vi "RILIS Narrow Band Scan Coordinator.vi"() -> ()   [LabVIEW 2013]
uses:
  RILIS Narrow Band Scan Coordinator States.ctl
panel:
  in  "Shared Variable Selection":enum16{"CRIS", "Test"}(ring)
  out "waveReadback":dbl format="%#.4f"
  in  "waveSet":dbl format="%.4f"
  out "Current State":T1
  in  "Find Center":bool
  out "Actual Wavenumber":dbl format="%#.4f"
  out "Loop Counter":i32
  in  "Stop Program":bool
  in  "Scanning Step Size":dbl format="%#.4f"
  in  "End of Scan Range":dbl format="%#.4f"
  in  "Start of Scan Range":dbl format="%#.4f"
  out "Measurement Complete":bool
  out "Averaging Active":bool
  out "isOK":bool
  in  "isNew":bool
  out "Linewidth Sweep Done":bool
  out "Moving to Setpoint":bool
  in  "Setpoint Wavenumber":dbl format="%.4f"
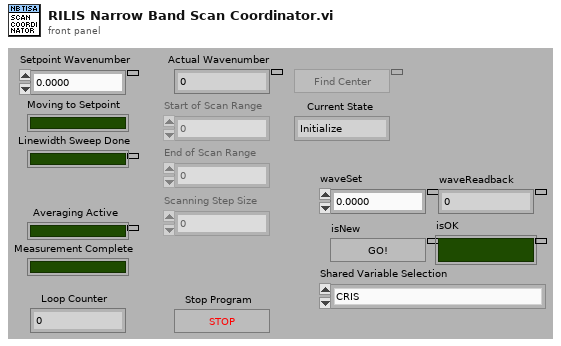
[diagram p1: front panel]
types:
  T1 = typedef "RILIS Narrow Band Scan Coordinator States.ctl" = enum16{"Initialize", "Idle", "Read Setpoint WN", "Check Setpoint WN", "Move to Setpoint WN", "Perform Sweep", "Wait for Ready", "Measurement in Progress", "Stop"}
  T2 = cluster{"Moving to Setpoint":bool, "Linewidth Sweep Done":bool, "Ready to Average":bool, "Averaging Active":bool, "Measurement Complete":bool, "Setpoint Wavenumber":dbl}
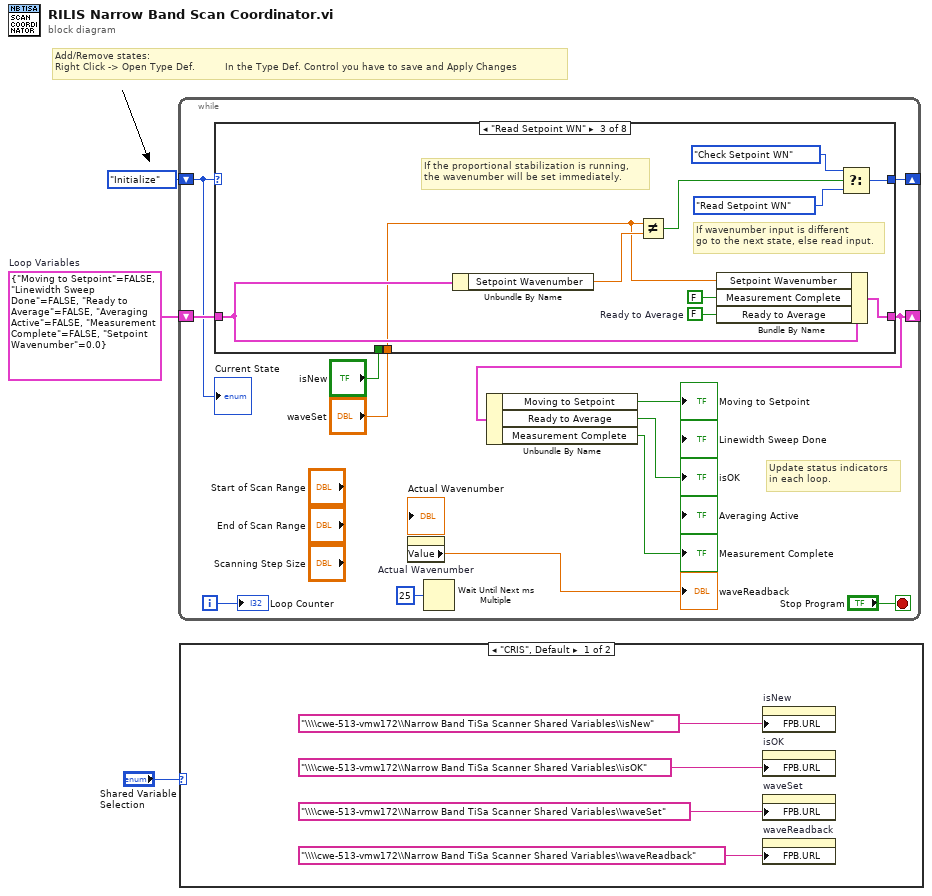
[diagram p0: block diagram]
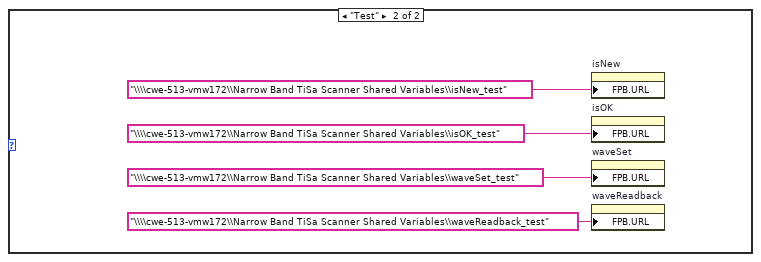
[diagram p2: hidden frame]
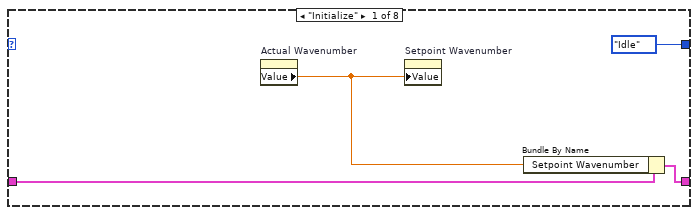
[diagram p3: hidden frame]
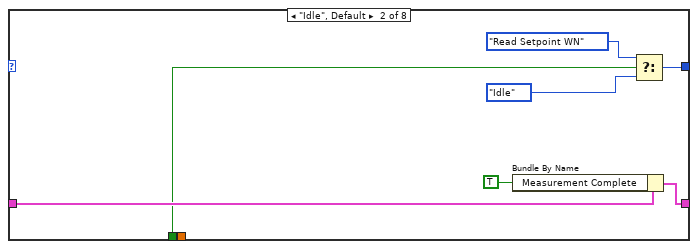
[diagram p4: hidden frame]
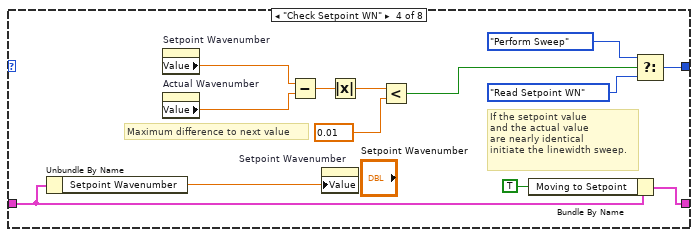
[diagram p5: hidden frame]
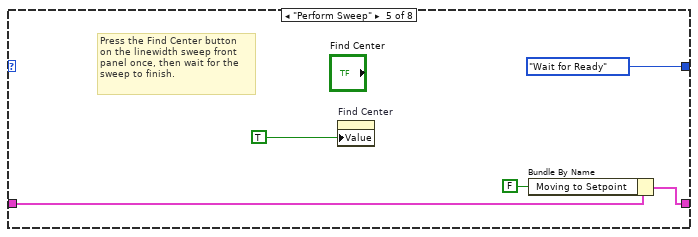
[diagram p6: hidden frame]
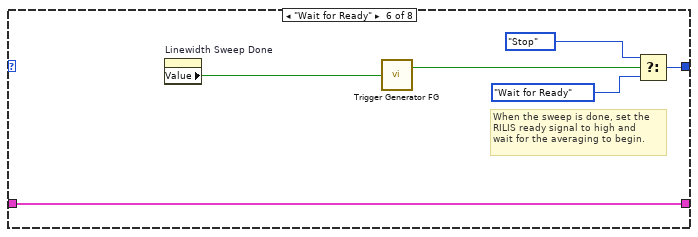
[diagram p7: hidden frame]
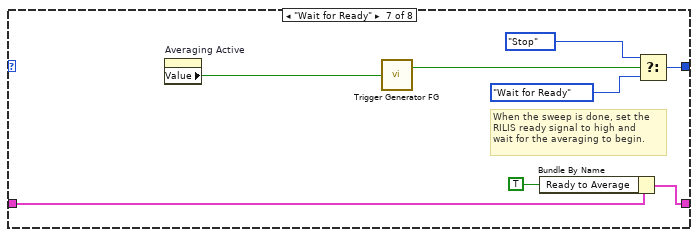
[diagram p8: hidden frame]
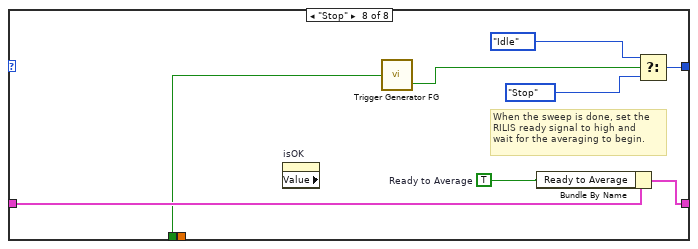
[diagram p9: hidden frame]
diagram:
  w2 = T2 {"Moving to Setpoint"=FALSE, "Linewidth Sweep Done"=FALSE, "Ready to Average"=FALSE, "Averaging Active"=FALSE, "Measurement Complete"=FALSE, "Setpoint Wavenumber"=0.0}  # Loop Variables
  # "Add/Remove states:\nRight Click -> Open Type Def.          In the Type Def. Control you have to save and Apply Changes"
  n1 = while {
    shift-right: [w13] -> _
    shift-left: RILIS_Narrow_Band_Scan_Coordinator_States."Initialize" ("NB Scan States") -> [w11]
    shift-right: [w10] -> _
    shift-left: w2 -> [w12]
    i -> [w15]
    stop <- "Stop Program" stop-if-true
    # "Update status indicators \nin each loop."
    n2 = case shown="\"Read Setpoint WN\"" w11 {
      tunnel: [RILIS_Narrow_Band_Scan_Coordinator_States."Idle" ("NB Scan States") w25 w37 w43 RILIS_Narrow_Band_Scan_Coordinator_States."Wait for Ready" ("NB Scan States") w59 w67 w75] -> w13
      tunnel: w12 -> [w19 w23 w32 w39 w52 w56 w63 w73]
      tunnel: [w18 w22 w31 w41 w51 w56 w62 w72] -> w10
      tunnel: "isNew" -> [_ w21 _ _ _ _ _ w70]
      tunnel: "waveSet" -> [_ _ w29 _ _ _ _ _]
      frame "Initialize" {
        n3 = property on="Actual Wavenumber" class="DigNum (strict)"() -> ("Value"=w17:dbl)  [unwired: 2 in, 2 out]
        n4 = property on="Setpoint Wavenumber" class="DigNum (strict)"("Value"=w17) -> ()  [unwired: 2 in, 2 out]
        n5 = Bundle By Name(cluster=w19, "Setpoint Wavenumber"=w17) -> (w18:T2)
      }
      frame "Idle", Default {
        n6 = Bundle By Name(cluster=w23, "Measurement Complete"=TRUE) -> (w22:T2)
        n7 = Select(t=RILIS_Narrow_Band_Scan_Coordinator_States."Read Setpoint WN" ("NB Scan States"), s=w21, f=RILIS_Narrow_Band_Scan_Coordinator_States."Idle" ("NB Scan States")) -> (s? t:f=w25:T1)
      }
      frame "Read Setpoint WN" {
        w28 = FALSE  # Ready to Average
        # "If wavenumber input is different\ngo to the next state, else read input."
        # "If the proportional stabilization is running, \nthe wavenumber will be set immediately."
        n8 = Unbundle By Name(w32) -> ("Setpoint Wavenumber"=w34:dbl)
        n9 = Not Equal?(x=w29, y=w34) -> (x != y?=w30:bool)
        n10 = Bundle By Name(cluster=w32, "Setpoint Wavenumber"=w29, "Measurement Complete"=FALSE, "Ready to Average"=w28) -> (w31:T2)
        n11 = Select(t=RILIS_Narrow_Band_Scan_Coordinator_States."Check Setpoint WN" ("NB Scan States"), s=w30, f=RILIS_Narrow_Band_Scan_Coordinator_States."Read Setpoint WN" ("NB Scan States")) -> (s? t:f=w37:T1)
      }
      frame "Check Setpoint WN" {
        # "Maximum difference to next value"
        # "If the setpoint value \nand the actual value\nare nearly identical \ninitiate the linewidth sweep."
        n12 = Unbundle By Name(w39) -> ("Setpoint Wavenumber"=w38:dbl)
        n13 = property on="Setpoint Wavenumber" class="DigNum (strict)"() -> ("Value"=w50:dbl)  [unwired: 2 in, 2 out]
        n14 = property on="Actual Wavenumber" class="DigNum (strict)"() -> ("Value"=w49:dbl)  [unwired: 2 in, 2 out]
        n15 = Subtract(x=w50, y=w49) -> (x-y=w48:dbl)
        n16 = property on="Setpoint Wavenumber" class="DigNum (strict)"("Value"=w38) -> ()  [unwired: 2 in, 2 out]
        n17 = Absolute Value(x=w48) -> (abs(x)=w47:dbl)
        n18 = Less?(x=w47, y=0.01) -> (x < y?=w42:bool)
        n19 = Bundle By Name(cluster=w39, "Moving to Setpoint"=TRUE) -> (w41:T2)
        n20 = Select(t=RILIS_Narrow_Band_Scan_Coordinator_States."Perform Sweep" ("NB Scan States"), s=w42, f=RILIS_Narrow_Band_Scan_Coordinator_States."Read Setpoint WN" ("NB Scan States")) -> (s? t:f=w43:T1)
      }
      frame "Perform Sweep" {
        # "Press the Find Center button \non the linewidth sweep front\npanel once, then wait for the \nsweep to finish."
        n21 = property on="Find Center" class="Bool (strict)"("Value"=TRUE) -> ()  [unwired: 2 in, 2 out]
        n22 = Bundle By Name(cluster=w52, "Moving to Setpoint"=FALSE) -> (w51:T2)
      }
      frame "Wait for Ready" {
        # "When the sweep is done, set the \nRILIS ready signal to high and \nwait for the averaging to begin."
        n23 = property on="Linewidth Sweep Done" class="Bool (strict)"() -> ("Value"=w58:bool)  [unwired: 2 in, 2 out]
        n24 = call "Trigger Generator FG.vi"("Boolean in"=w58) -> ("Rising Trigger out"=w57:bool)  [unwired: 1 out]
        n25 = Select(t=RILIS_Narrow_Band_Scan_Coordinator_States."Stop" ("NB Scan States"), s=w57, f=RILIS_Narrow_Band_Scan_Coordinator_States."Wait for Ready" ("NB Scan States")) -> (s? t:f=w59:T1)
      }
      frame "Wait for Ready" {
        # "When the sweep is done, set the \nRILIS ready signal to high and \nwait for the averaging to begin."
        n26 = property on="Averaging Active" class="Bool (strict)"() -> ("Value"=w65:bool)  [unwired: 2 in, 2 out]
        n27 = call "Trigger Generator FG.vi"("Boolean in"=w65) -> ("Rising Trigger out"=w66:bool)  [unwired: 1 out]
        n28 = Bundle By Name(cluster=w63, "Ready to Average"=TRUE) -> (w62:T2)
        n29 = Select(t=RILIS_Narrow_Band_Scan_Coordinator_States."Stop" ("NB Scan States"), s=w66, f=RILIS_Narrow_Band_Scan_Coordinator_States."Wait for Ready" ("NB Scan States")) -> (s? t:f=w67:T1)
      }
      frame "Stop" {
        w71 = TRUE  # Ready to Average
        # "When the sweep is done, set the \nRILIS ready signal to high and \nwait for the averaging to begin."
        n30 = property on="isOK" class="Bool (strict)" props=["Value"]() -> ()  [unwired: 2 in, 3 out]
        n31 = call "Trigger Generator FG.vi"("Boolean in"=w70) -> ("Falling Trigger out"=w74:bool)  [unwired: 1 out]
        n32 = Bundle By Name(cluster=w73, "Ready to Average"=w71) -> (w72:T2)
        n33 = Select(t=RILIS_Narrow_Band_Scan_Coordinator_States."Idle" ("NB Scan States"), s=w74, f=RILIS_Narrow_Band_Scan_Coordinator_States."Stop" ("NB Scan States")) -> (s? t:f=w75:T1)
      }
    }
    n34 = property on="Actual Wavenumber" class="DigNum (strict)"() -> ("Value"=→"waveReadback":dbl)  [unwired: 2 in, 2 out]
    n35 = Wait Until Next ms Multiple(millisecond multiple=u32 25) -> ()  [unwired: 1 out]
    n36 = Unbundle By Name(w10) -> ("Moving to Setpoint"=→"Moving to Setpoint":bool, "Ready to Average"=→"isOK":bool, "Measurement Complete"=→"Measurement Complete":bool)
    "Loop Counter" <- w15
    "Current State" <- w11
  }
  n37 = case shown="\"CRIS\", Default" "Shared Variable Selection" {
    frame "CRIS", Default {
      n38 = property on="isNew" class="Bool (strict)"("FPB.URL"="\\\\cwe-513-vmw172\\Narrow Band TiSa Scanner Shared Variables\\isNew") -> ()  [unwired: 2 in, 2 out]
      n39 = property on="isOK" class="Bool (strict)"("FPB.URL"="\\\\cwe-513-vmw172\\Narrow Band TiSa Scanner Shared Variables\\isOK") -> ()  [unwired: 2 in, 2 out]
      n40 = property on="waveSet" class="DigNum (strict)"("FPB.URL"="\\\\cwe-513-vmw172\\Narrow Band TiSa Scanner Shared Variables\\waveSet") -> ()  [unwired: 2 in, 2 out]
      n41 = property on="waveReadback" class="DigNum (strict)"("FPB.URL"="\\\\cwe-513-vmw172\\Narrow Band TiSa Scanner Shared Variables\\waveReadback") -> ()  [unwired: 2 in, 2 out]
    }
    frame "Test" {
      n42 = property on="isNew" class="Bool (strict)"("FPB.URL"="\\\\cwe-513-vmw172\\Narrow Band TiSa Scanner Shared Variables\\isNew_test") -> ()  [unwired: 2 in, 2 out]
      n43 = property on="isOK" class="Bool (strict)"("FPB.URL"="\\\\cwe-513-vmw172\\Narrow Band TiSa Scanner Shared Variables\\isOK_test") -> ()  [unwired: 2 in, 2 out]
      n44 = property on="waveSet" class="DigNum (strict)"("FPB.URL"="\\\\cwe-513-vmw172\\Narrow Band TiSa Scanner Shared Variables\\waveSet_test") -> ()  [unwired: 2 in, 2 out]
      n45 = property on="waveReadback" class="DigNum (strict)"("FPB.URL"="\\\\cwe-513-vmw172\\Narrow Band TiSa Scanner Shared Variables\\waveReadback_test") -> ()  [unwired: 2 in, 2 out]
    }
  }
